vi "io.az-pos.vi"(11 "Cluster":T1) -> (3 "Numeric":fxp<+/-,32,2>)   [LabVIEW 2019]
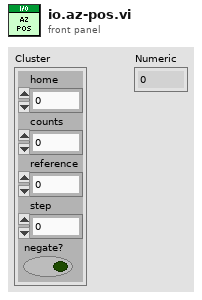
[diagram p1: front panel]
types:
  T1 = cluster{"home":fxp<+/-,32,2>, "counts":u64, "reference":u64, "step":u64, "negate?":bool}
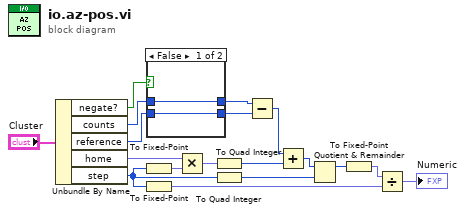
[diagram p0: block diagram]
diagram:
  n1 = Unbundle By Name("Cluster") -> ("negate?"=w14:bool, "counts"=w15:u64, "reference"=w16:u64, "home"=w17:fxp<+/-,32,2>, "step"=w18:u64)
  n2 = To Fixed-Point(number=w18) -> (fixed-point=w6:fxp<+,64,64>)  [unwired: 1 in]
  n3 = To Fixed-Point(number=w18) -> (fixed-point=w4:fxp<+/-,64,64>)  [unwired: 1 in]
  n4 = case shown="False" w14 {
    tunnel: [w20 w22] -> w11
    tunnel: w15 -> [w20 w21]
    tunnel: [w19 w21] -> w12
    tunnel: w16 -> [w19 w22]
    frame False {
    }
    frame True {
    }
  }
  n5 = Multiply(x=w17, y=w6) -> (x*y=w7:fxp<+/-,64,64>)
  n6 = To Quad Integer(1:w7) -> (0:w9:i64)
  n7 = To Quad Integer(1:w18) -> (0:w1:i64)
  n8 = Subtract(x=w11, y=w12) -> (x-y=w8:i64)
  n9 = Add(x=w8, y=w9) -> (x+y=w10:i64)
  n10 = Quotient & Remainder(x=w10, y=w1) -> (x-y*floor(x/y)=w3:i64)  [unwired: 1 out]
  n11 = To Fixed-Point(number=w3) -> (fixed-point=w2:fxp<+/-,64,64>)  [unwired: 1 in]
  n12 = Divide(x=w2, y=w4) -> (x/y=→"Numeric":fxp<+/-,32,2>)
